vi "InsertNode.vi"(6 "Insert Search":T1={"InsertIfEmpty"=TRUE, "Insert After"=TRUE, "InsertIfNotFound"=FALSE}, 8 "error in (no error)":errorcluster, 9 "position":T2=enum."Back", 10 "ToInsert":refnum<data-value>, 11 "LinkedList in":refnum<class "LinkedList.lvclass">) -> (0 "error out":errorcluster, 1 "ignored":bool, 3 "LinkedList out":refnum<class "LinkedList.lvclass">)   [LabVIEW 2013, in "LinkedList.lvclass"]
doc: "Inserts a node into the linked list based on the position. The search of where to insert starts at the root and move to the back. Override the IsSearchGoalNode.vi to make the insertion point searchable."
uses:
  LinkedList.lvclass
  position.ctl
  LLNode/LLNode.lvclass
  InsertSearchOptions.ctl
  LinkedList.lvclass/LinkedList.ctl
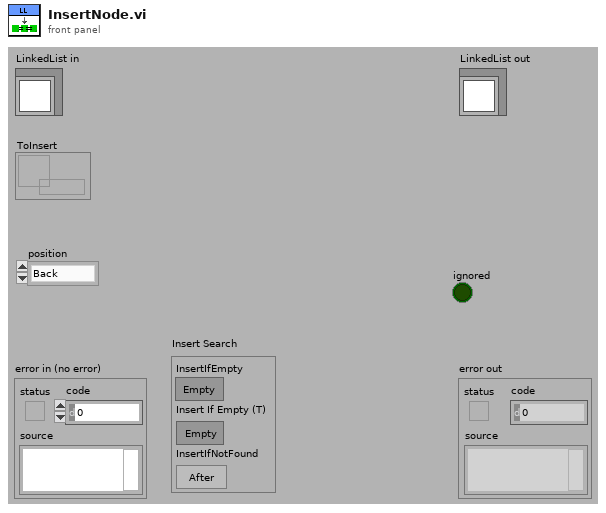
[diagram p1: front panel]
types:
  T1 = typedef "LinkedList.lvclass/InsertSearchOptions.ctl" = cluster{"InsertIfEmpty":bool, "Insert After":bool, "InsertIfNotFound":bool}
  T2 = typedef "LinkedList.lvclass/position.ctl" = enum16{"Front", "Back", "Search"}
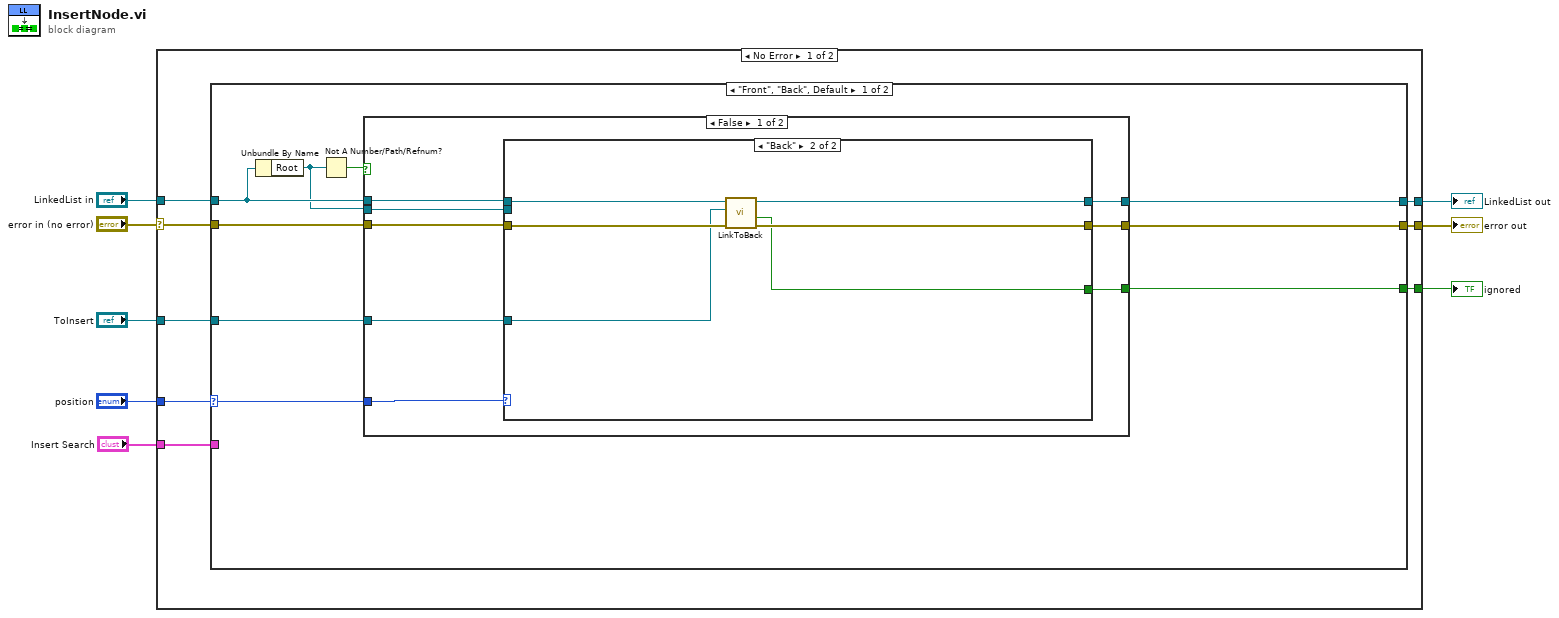
[diagram p0: block diagram]
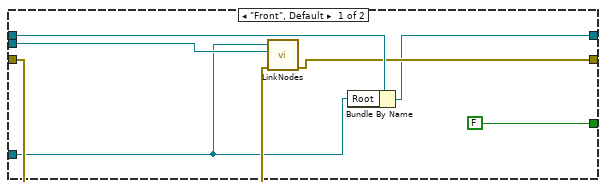
[diagram p2: hidden frame]
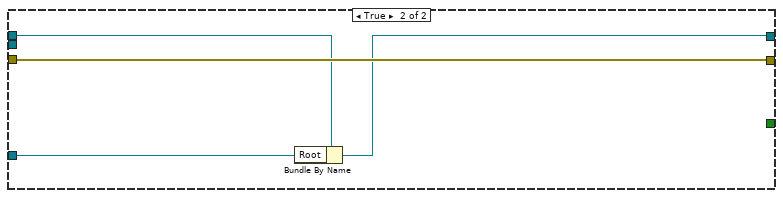
[diagram p3: hidden frame]
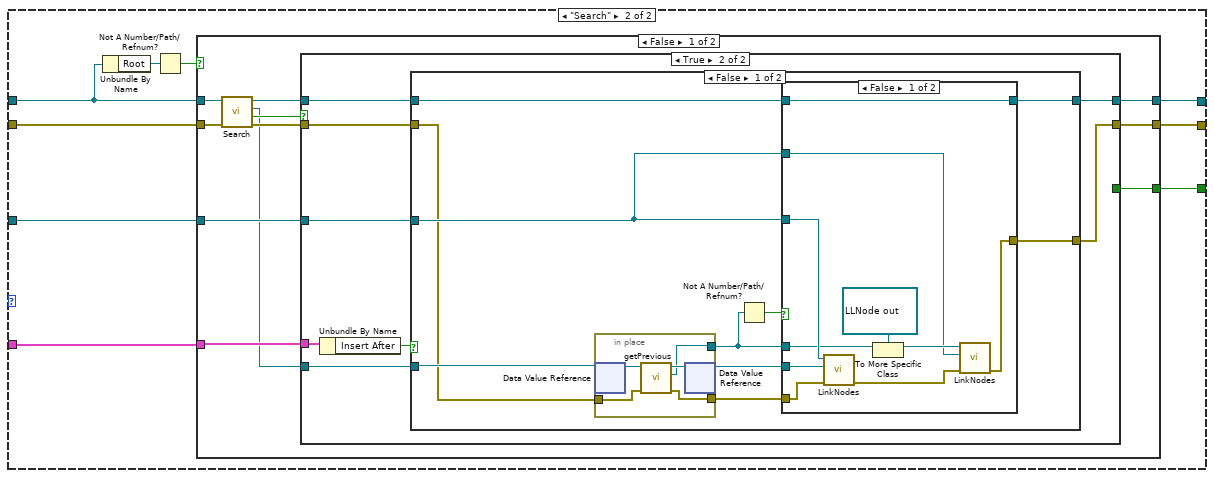
[diagram p4: hidden frame]
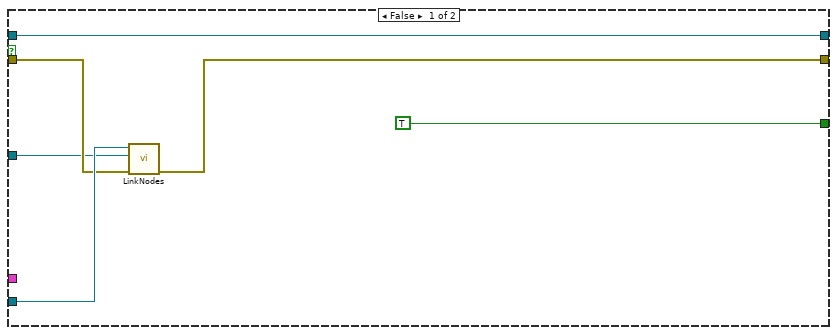
[diagram p5: hidden frame]
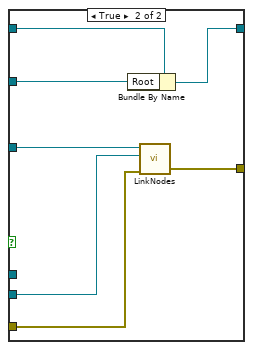
[diagram p6: hidden frame]
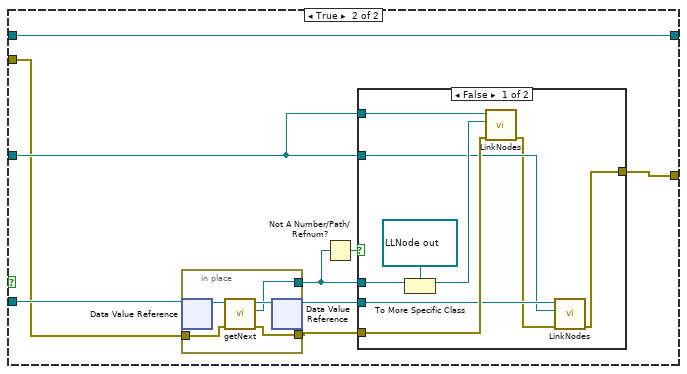
[diagram p7: hidden frame]
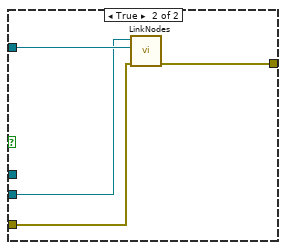
[diagram p8: hidden frame]
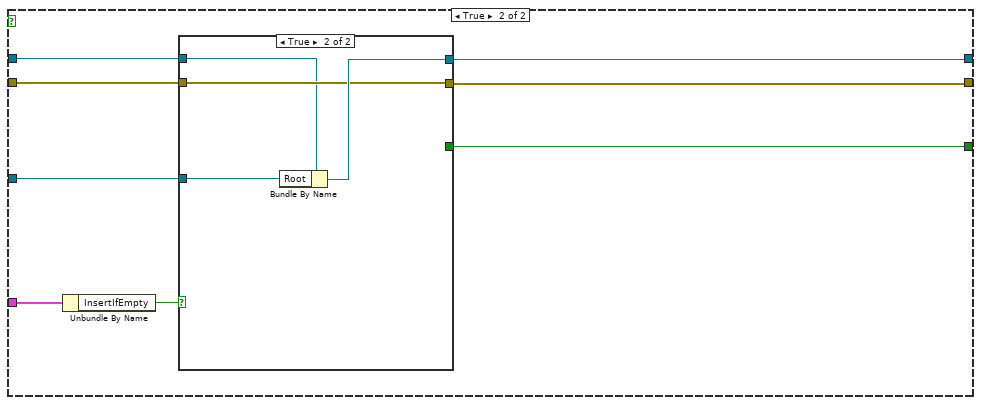
[diagram p9: hidden frame]
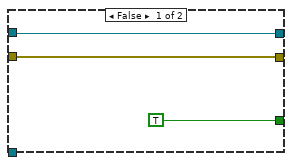
[diagram p10: hidden frame]
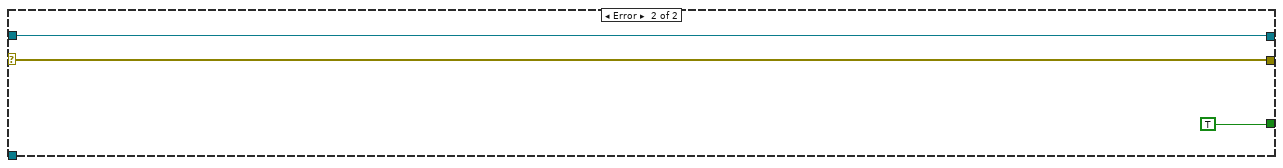
[diagram p11: hidden frame]
diagram:
  n1 = case shown="No Error" "error in (no error)" {
    selector: "error in (no error)" -> [w11 w161]
    tunnel: [w9 w161] -> w7
    tunnel: [w10 w160] -> w6
    tunnel: "LinkedList in" -> [w12 w160]
    tunnel: "ToInsert" -> [w13 _]
    tunnel: "position" -> [w16 _]
    tunnel: [w15 TRUE] -> w2
    tunnel: "Insert Search" -> [w14 _]
    frame No Error {
      n2 = case shown="\"Front\", \"Back\", Default" w16 {
        selector: w16 -> [w25 _]
        tunnel: w12 -> [w19 w54]
        tunnel: [w22 w59] -> w10
        tunnel: [w21 w58] -> w9
        tunnel: [w24 w57] -> w15
        tunnel: w13 -> [w23 w55]
        tunnel: w11 -> [w18 w53]
        tunnel: w14 -> [_ w56]
        frame "Front", "Back", Default {
          n3 = Unbundle By Name(w19) -> ("Root"=w17:refnum<data-value>)
          n4 = Not A Number/Path/Refnum?(number/path/refnum=w17) -> (NaN/Path/Refnum?=w20:bool)
          n5 = case shown="False" w20 {
            tunnel: w18 -> [w32 w50]
            tunnel: w19 -> [w27 w48]
            tunnel: w23 -> [w30 w49]
            tunnel: [w26 w47] -> w22
            tunnel: w17 -> [w33 _]
            tunnel: [w31 w50] -> w21
            tunnel: w25 -> [w28 _]
            tunnel: [w29 _] -> w24
            frame False {
              n6 = case shown="\"Back\"" w28 {
                tunnel: w33 -> [w39 _]
                tunnel: w32 -> [w35 w45]
                tunnel: [w37 w44] -> w31
                tunnel: w30 -> [w34 w42]
                tunnel: [FALSE ("ignored") w41] -> w29
                tunnel: w27 -> [w38 w46]
                tunnel: [w36 w43] -> w26
                frame "Front", Default {
                  n7 = call "LinkNodes.vi"("error in (no error)"=w35, "NextNode in"=w39, "PreviousNode in"=w34) -> ("error out"=w37:errorcluster)  [unwired: 6 in, 2 out]
                  n8 = Bundle By Name(cluster=w38, "Root"=w34) -> (w36:refnum<class "LinkedList.lvclass">)
                }
                frame "Back" {
                  n9 = call "LinkToBack.vi"("error in (no error)"=w45, "newBackNode"=w42, "LinkedList in"=w46) -> ("error out"=w44:errorcluster, "ignored"=w41:bool, "LinkedList out"=w43:refnum<class "LinkedList.lvclass">)  [unwired: 6 in]
                }
              }
            }
            frame True {
              n10 = Bundle By Name(cluster=w48, "Root"=w49) -> (w47:refnum<class "LinkedList.lvclass">)
            }
          }
        }
        frame "Search" {
          n11 = Unbundle By Name(w54) -> ("Root"=w51:refnum<data-value>)
          n12 = Not A Number/Path/Refnum?(number/path/refnum=w51) -> (NaN/Path/Refnum?=w52:bool)
          n13 = case shown="False" w52 {
            tunnel: w54 -> [w65 w150]
            tunnel: w53 -> [w63 w147]
            tunnel: [w66 w145] -> w59
            tunnel: [w69 w146] -> w58
            tunnel: [w67 w144] -> w57
            tunnel: w56 -> [w68 w151]
            tunnel: w55 -> [w70 w148]
            frame False {
              n14 = call "Search.vi"("error in (no error)"=w63, "LinkedList in"=w65) -> ("error out"=w62:errorcluster, "found"=w61:bool, "Node"=w60:refnum<data-value>, "LinkedList out"=w64:refnum<class "LinkedList.lvclass">)  [unwired: 6 in]
              n15 = case shown="True" w61 {
                tunnel: w60 -> [w74 w80]
                tunnel: w70 -> [w72 w81]
                tunnel: w62 -> [w73 w82]
                tunnel: [w71 w79] -> w69
                tunnel: w68 -> [_ w84]
                tunnel: [TRUE _] -> w67
                tunnel: w64 -> [w75 w78]
                tunnel: [w75 w77] -> w66
                frame False {
                  n16 = call "LinkNodes.vi"("error in (no error)"=w73, "NextNode in"=w72, "PreviousNode in"=w74) -> ("error out"=w71:errorcluster)  [unwired: 6 in, 2 out]
                }
                frame True {
                  n17 = Unbundle By Name(w84) -> ("Insert After"=w83:bool)
                  n18 = case shown="False" w83 {
                    tunnel: w82 -> [w85 w117]
                    tunnel: w81 -> [w86 w118]
                    tunnel: w80 -> [w94 w125]
                    tunnel: [w91 w122] -> w79
                    tunnel: w78 -> [w90 w121]
                    tunnel: [w89 w121] -> w77
                    frame False {
                      n19 = in-place {
                        in-place-border: [w114] -> w87
                        in-place-border: w85 -> [w113]
                        in-place-border: [w112] -> w92
                        n20 = in-place-dvr #1(w94) -> (w116:refnum<class "LLNode.lvclass">)  [unwired: 1 out]
                        n21 = call "getPrevious.vi"("error in (no error)"=w113, "LLNode in"=w116) -> ("error out"=w112:errorcluster, "previous"=w114:refnum<data-value>, "LLNode out"=w115:refnum<class "LLNode.lvclass">)  [unwired: 7 in]
                        n22 = in-place-dvr #1(w115) -> (w93:refnum<data-value>)  [unwired: 1 out]
                      }
                      n23 = Not A Number/Path/Refnum?(number/path/refnum=w87) -> (NaN/Path/Refnum?=w88:bool)
                      n24 = case shown="False" w88 {
                        tunnel: w86 -> [w96 w106]
                        tunnel: w86 -> [w101 w110]
                        tunnel: w93 -> [w103 w111]
                        tunnel: w92 -> [w102 w109]
                        tunnel: w87 -> [w100 _]
                        tunnel: [w97 w108] -> w91
                        tunnel: w90 -> [w104 w107]
                        tunnel: [w104 w105] -> w89
                        frame False {
                          n25 = call "LinkNodes.vi"("error in (no error)"=w102, "NextNode in"=w103, "PreviousNode in"=w101) -> ("error out"=w95:errorcluster)  [unwired: 6 in, 2 out]
                          n26 = To More Specific Class(target class=refnum<data-value> refnum ("ToInsert"), reference=w100) -> (specific class reference=w98:refnum<data-value>)  [unwired: 1 in, 1 out]
                          n27 = call "LinkNodes.vi"("error in (no error)"=w95, "NextNode in"=w96, "PreviousNode in"=w98) -> ("error out"=w97:errorcluster)  [unwired: 6 in, 2 out]
                        }
                        frame True {
                          n28 = Bundle By Name(cluster=w107, "Root"=w106) -> (w105:refnum<class "LinkedList.lvclass">)
                          n29 = call "LinkNodes.vi"("error in (no error)"=w109, "NextNode in"=w111, "PreviousNode in"=w110) -> ("error out"=w108:errorcluster)  [unwired: 6 in, 2 out]
                        }
                      }
                    }
                    frame True {
                      n30 = in-place {
                        in-place-border: [w141] -> w119
                        in-place-border: w117 -> [w140]
                        in-place-border: [w139] -> w123
                        n31 = in-place-dvr #2(w125) -> (w143:refnum<class "LLNode.lvclass">)  [unwired: 1 out]
                        n32 = call "getNext.vi"("error in (no error)"=w140, "LLNode in"=w143) -> ("error out"=w139:errorcluster, "next"=w141:refnum<data-value>, "LLNode out"=w142:refnum<class "LLNode.lvclass">)  [unwired: 7 in]
                        n33 = in-place-dvr #2(w142) -> (w124:refnum<data-value>)  [unwired: 1 out]
                      }
                      n34 = Not A Number/Path/Refnum?(number/path/refnum=w119) -> (NaN/Path/Refnum?=w120:bool)
                      n35 = case shown="False" w120 {
                        tunnel: w118 -> [w128 w138]
                        tunnel: w118 -> [w134 _]
                        tunnel: w119 -> [w133 _]
                        tunnel: w124 -> [w129 w137]
                        tunnel: w123 -> [w130 w136]
                        tunnel: [w126 w135] -> w122
                        frame False {
                          n36 = To More Specific Class(target class=refnum<data-value> refnum ("ToInsert"), reference=w133) -> (specific class reference=w131:refnum<data-value>)  [unwired: 1 in, 1 out]
                          n37 = call "LinkNodes.vi"("error in (no error)"=w130, "NextNode in"=w131, "PreviousNode in"=w134) -> ("error out"=w127:errorcluster)  [unwired: 6 in, 2 out]
                          n38 = call "LinkNodes.vi"("error in (no error)"=w127, "NextNode in"=w128, "PreviousNode in"=w129) -> ("error out"=w126:errorcluster)  [unwired: 6 in, 2 out]
                        }
                        frame True {
                          n39 = call "LinkNodes.vi"("error in (no error)"=w136, "NextNode in"=w138, "PreviousNode in"=w137) -> ("error out"=w135:errorcluster)  [unwired: 6 in, 2 out]
                        }
                      }
                    }
                  }
                }
              }
            }
            frame True {
              n40 = Unbundle By Name(w151) -> ("InsertIfEmpty"=w149:bool)
              n41 = case shown="True" w149 {
                tunnel: w150 -> [w152 w155]
                tunnel: w148 -> [_ w156]
                tunnel: w147 -> [w153 w157]
                tunnel: [w153 w157] -> w146
                tunnel: [w152 w158] -> w145
                tunnel: [TRUE _] -> w144
                frame False {
                }
                frame True {
                  n42 = Bundle By Name(cluster=w155, "Root"=w156) -> (w158:refnum<class "LinkedList.lvclass">)
                }
              }
            }
          }
        }
      }
    }
    frame Error {
    }
  }
  "error out" <- w7
  "LinkedList out" <- w6
  "ignored" <- w2
